vi "linie XY major.vi"(6 "Y Scale.Grid Colors:Major Color":u32, 10 "error in (no error)":errorcluster, 11 "WaveformGraph in":refnum<vi>) -> (2 "error out":errorcluster)   [LabVIEW 2014]
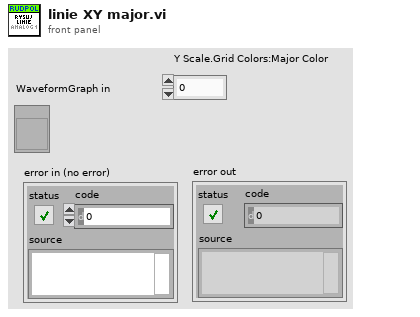
[diagram p1: front panel]
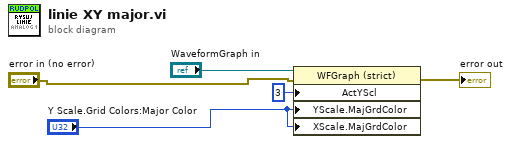
[diagram p0: block diagram]
diagram:
  n1 = property class="WFGraph (strict)"(reference="WaveformGraph in", error in="error in (no error)", "ActYScl"=3 ("Active Y Scale"), "YScale.MajGrdColor"="Y Scale.Grid Colors:Major Color", "XScale.MajGrdColor"="Y Scale.Grid Colors:Major Color") -> (error out=→"error out":errorcluster)  [unwired: 1 out]
